vi "Leggi file testi.vi"(3 "Lunghezza":i32, 4 "Numero riga":i32) -> (0 "Array testo":string[](array[string]), 1 "Testo":string)   [LabVIEW 2022 SP3]
uses:
  Labview/Globali.vi
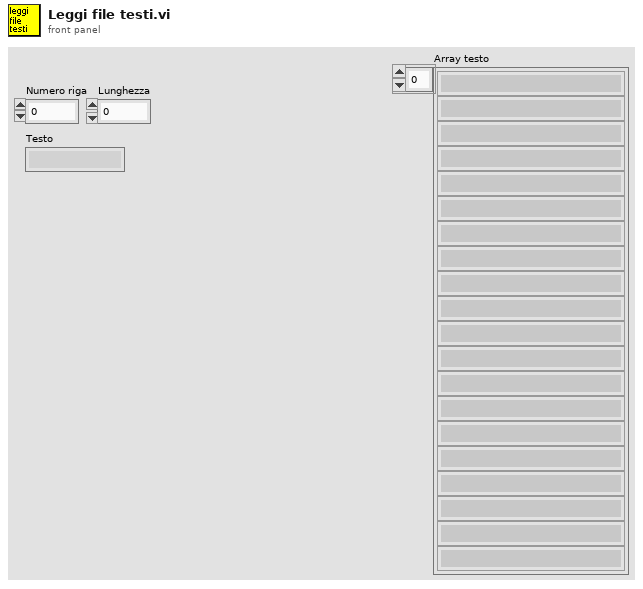
[diagram p1: front panel]
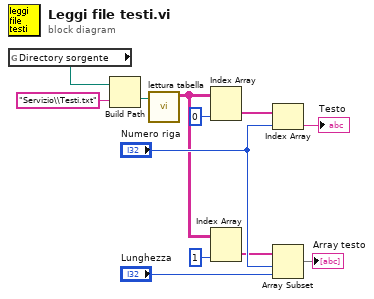
[diagram p0: block diagram]
diagram:
  n1 = global read "Globali.vi" "Directory sorgente"() -> (w8:path)
  n2 = Build Path(base path=w8, name or relative path="Servizio\\Testi.txt") -> (appended path=w11:path)
  n3 = call "lettura tabella.vi"("file path (dialog if empty)"=w11) -> ("all rows"=w1:string[][])  [unwired: 6 in, 4 out]
  n4 = Index Array(array=w1, index (col)=0 ("index (row)")) -> (element=w3:string[])  [unwired: 1 in]
  n5 = Index Array(array=w1, index (col)=1 ("disabled index (col)")) -> (element=w2:string[])  [unwired: 1 in]
  n6 = Index Array(array=w3, index="Numero riga") -> (element=→"Testo":string)
  n7 = Array Subset(array=w2, index="Numero riga", length="Lunghezza") -> (→"Array testo":string[])
